vi "Check Timeout.vi"(8 "error in (no error)":errorcluster, 11 "Lamp in":refnum<class "Lamp.lvclass">) -> (0 "error out":errorcluster, 3 "Lamp out":refnum<class "Lamp.lvclass">)   [LabVIEW 2016, in "Lamp.lvclass"]
uses:
  Lamp.lvclass
  Lamp.lvclass/Lamp.ctl
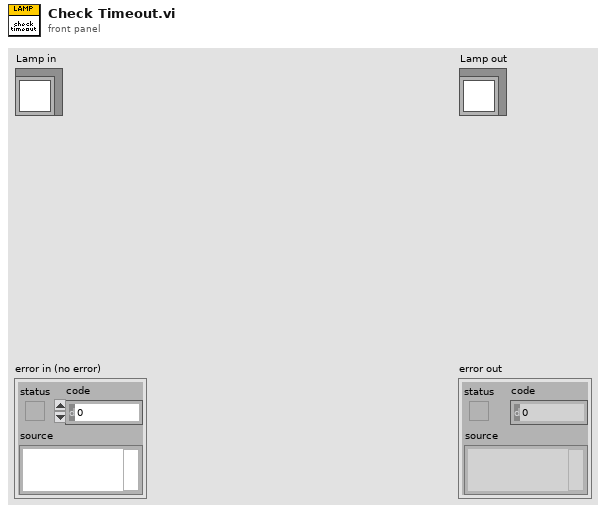
[diagram p1: front panel]
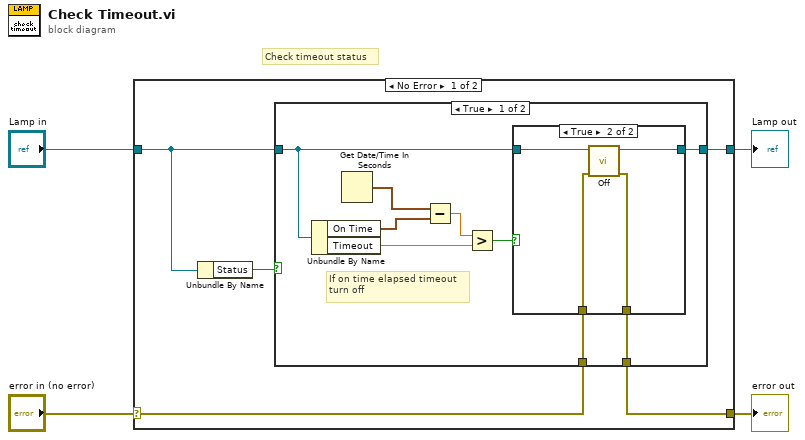
[diagram p0: block diagram]
diagram:
  # "Check timeout status"
  n1 = case shown="No Error" "error in (no error)" {
    selector: "error in (no error)" -> [w6 w28]
    tunnel: [w5 w28] -> w3
    tunnel: [w7 w27] -> w1
    tunnel: "Lamp in" -> [w8 w27]
    frame No Error {
      n2 = Unbundle By Name(w8) -> ("Status"=w9:bool)
      n3 = case shown="True" w9 {
        tunnel: w8 -> [w13 w26]
        tunnel: [w12 w26] -> w7
        tunnel: w6 -> [w11 w25]
        tunnel: [w10 w25] -> w5
        frame True {
          # "If on time elapsed timeout\nturn off"
          n4 = Unbundle By Name(w13) -> ("On Time"=w17:timestamp, "Timeout"=w15:dbl)
          n5 = Get Date/Time In Seconds() -> (seconds since 1Jan1904=w18:timestamp)
          n6 = Subtract(x=w18, y=w17) -> (x-y=w16:dbl)
          n7 = Greater?(x=w16, y=w15) -> (0:w14:bool)
          n8 = case shown="True" w14 {
            tunnel: w13 -> [w20 w24]
            tunnel: [w20 w23] -> w12
            tunnel: w11 -> [w19 w22]
            tunnel: [w19 w21] -> w10
            frame False {
            }
            frame True {
              n9 = call-dynamic "Off.vi"("error in (no error)"=w22, "Lamp in"=w24) -> ("error out"=w21:errorcluster, "Lamp out"=w23:refnum<class "Lamp.lvclass">)  [unwired: 8 in]
            }
          }
        }
        frame False {
        }
      }
    }
    frame Error {
    }
  }
  "error out" <- w3
  "Lamp out" <- w1
